vi "Get Monkeys.vi"(11 "Array in":string[](array[string])) -> (2 "Least Common Multiple":u64, 3 "Monkeys":T1(array[cluster]))   [LabVIEW 2021]
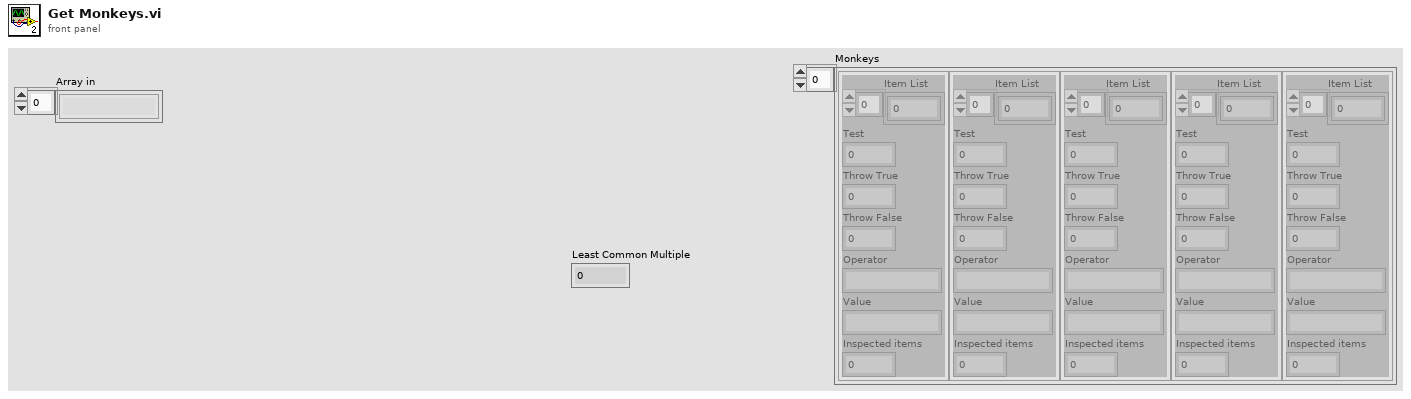
[diagram p1: front panel]
types:
  T1 = cluster{"Item List":u64[], "Test":u64, "Throw True":u64, "Throw False":u64, "Operator":string, "Value":string, "Inspected items":u64}[]
  T2 = cluster{"Item List":u64[], "Test":u64, "Throw True":u64, "Throw False":u64, "Operator":string, "Value":string, "Inspected items":u64}
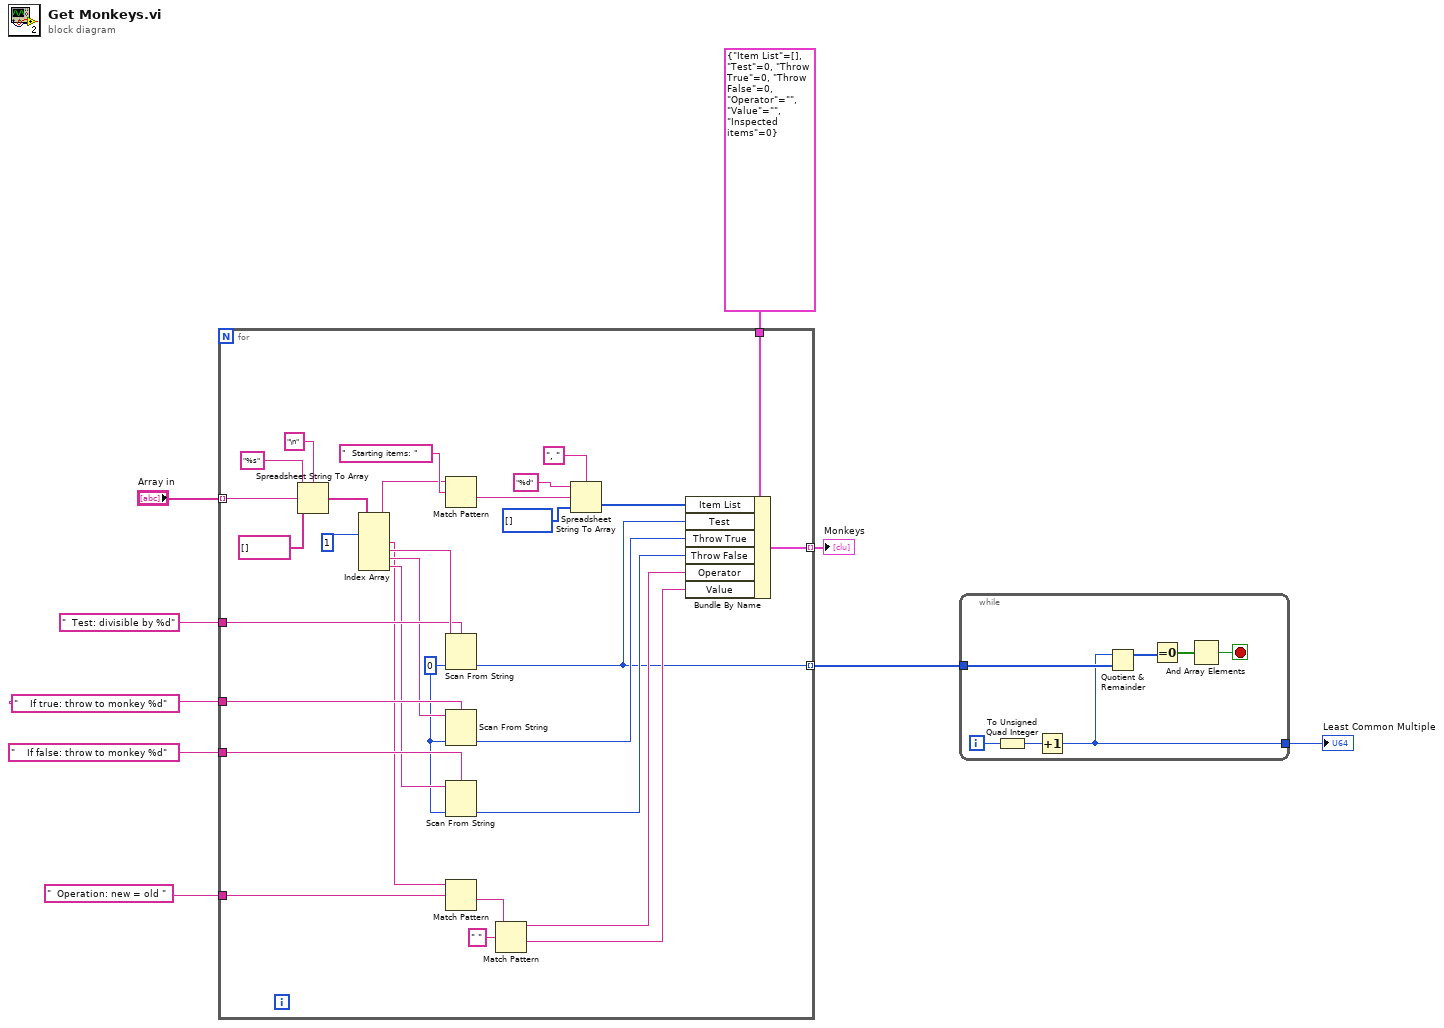
[diagram p0: block diagram]
diagram:
  n1 = for {
    tunnel: "Array in" -> [w40] mode=indexing
    tunnel: "  Test: divisible by %d" ("format string") -> [w31]
    tunnel: "    If true: throw to monkey %d" ("format string") -> [w30]
    tunnel: "    If false: throw to monkey %d" ("format string") -> [w28]
    tunnel: T2 {"Item List"=[], "Test"=0, "Throw True"=0, "Throw False"=0, "Operator"="", "Value"="", "Inspected items"=0} -> [w26]
    tunnel: [w21] -> w3 mode=indexing
    tunnel: "  Operation: new = old " ("format string") -> [w16]
    tunnel: [w10] -> w2 mode=indexing
    w25 = u64 0 ("default value 1")
    n2 = Spreadsheet String To Array(delimiter (Tab)="\n", format string="%s", spreadsheet string=w40, array type (2D Dbl)=string[] []) -> (array=w38:string[])
    n3 = Index Array(array=w38, index #1=1 ("index")) -> (element #1=w17:string, element #2=w15:string, element #3=w33:string, element #4=w29:string, element #5=w27:string)  [unwired: 4 in]
    n4 = Match Pattern(string=w17, regular expression="  Starting items: " ("format string")) -> (after substring=w34:string)  [unwired: 1 in, 3 out]
    n5 = Scan From String(format string=w31, input string=w33, default 1=w25) -> (output 1=w10:u64)  [unwired: 2 in, 3 out]
    n6 = Scan From String(format string=w30, input string=w29, default 1=w25) -> (output 1=w24:u64)  [unwired: 2 in, 3 out]
    n7 = Scan From String(format string=w28, input string=w27, default 1=w25) -> (output 1=w23:u64)  [unwired: 2 in, 3 out]
    n8 = Match Pattern(string=w15, regular expression=w16) -> (after substring=w14:string)  [unwired: 1 in, 3 out]
    n9 = Match Pattern(string=w14, regular expression=" ") -> (before substring=w12:string, after substring=w11:string)  [unwired: 1 in, 2 out]
    n10 = Spreadsheet String To Array(delimiter (Tab)=", ", format string="%d", spreadsheet string=w34, array type (2D Dbl)=u64[] []) -> (array=w22:u64[])
    n11 = Bundle By Name(cluster=w26, "Item List"=w22, "Test"=w10, "Throw True"=w24, "Throw False"=w23, "Operator"=w12, "Value"=w11) -> (w21:T2)
  }
  "Monkeys" <- w3
  n12 = while {
    tunnel: w2 -> [w43]
    tunnel: [w42] -> w1
    i -> [w47]
    stop <- w44 stop-if-true
    n13 = To Unsigned Quad Integer(1:w47) -> (0:w41:u64)
    n14 = Increment(x=w41) -> (x+1=w42:u64)
    n15 = Quotient & Remainder(x=w42, y=w43) -> (x-y*floor(x/y)=w46:u64[])  [unwired: 1 out]
    n16 = Equal To 0?(x=w46) -> (x = 0?=w45:bool[])
    n17 = And Array Elements(Boolean array=w45) -> (logical AND=w44:bool)
  }
  "Least Common Multiple" <- w1
